vi "Launcher.vi"() -> ()   [LabVIEW 2020]
uses:
  UI Actor.lvclass
  C:/Program Files (x86)/National Instruments/LabVIEW 2020/vi.lib/ActorFramework/Actor/Actor.lvclass
  UI Actor.lvclass/UI Actor.ctl
  Write Products.vi
  Write Coins.vi
  <vilib>/ActorFramework/Actor/Actor.lvclass
panel:
  in  "Coins":enum16{"USD", "MXN"}(ring)
  in  "Products":enum16{"Nestle", "Coca Cola"}(ring)
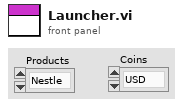
[diagram p1: front panel]
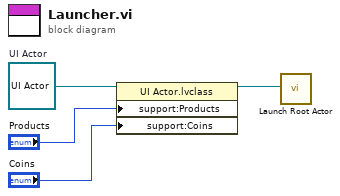
[diagram p0: block diagram]
diagram:
  w4 = refnum<class "UI Actor.lvclass"> refnum  # UI Actor
  n1 = property class="UI Actor.lvclass"(reference=w4, "support:Products"="Products", "support:Coins"="Coins") -> (reference out=w3:refnum<class "UI Actor.lvclass">)  [unwired: 1 in, 1 out]
  n2 = call <vilib>:"Launch Root Actor.vi"("Actor"=w3) -> ()  [unwired: 9 in, 2 out]
